vi "Corr Digitizer to Meas Folder.vi"(8 "error in":errorcluster, 10 "measurement root path":path, 11 "digitizer corr in":T1) -> (0 "error out":errorcluster, 3 "digitizer corr out":T1)   [LabVIEW 2020]
doc: "This VI will copy all digitizer corrections related folders to the measurement folder."
uses:
  Corr Digitizers.ctl
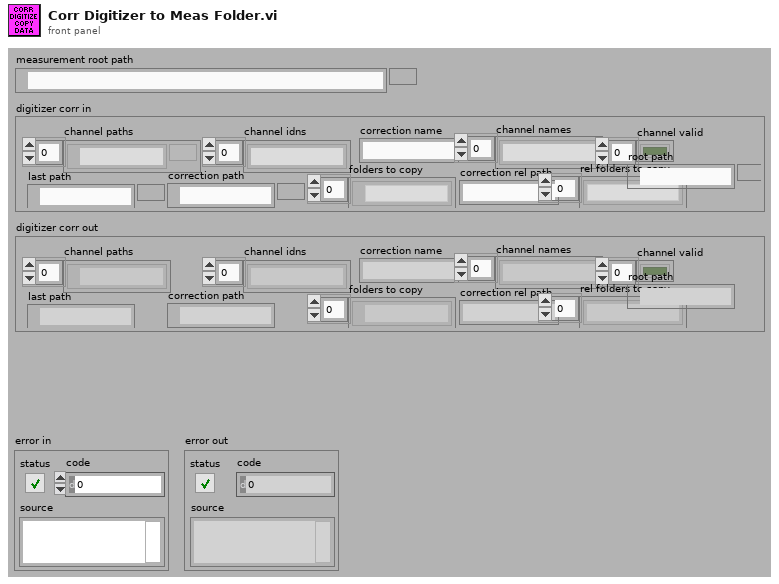
[diagram p1: front panel]
types:
  T1 = typedef "Corr Digitizers.ctl" = cluster{"last path":path, "channel paths":path[], "channel idns":string[], "correction name":string, "channel names":string[], "folders to copy":path[], "channel valid":bool[], "correction path":path, "correction rel path":string, "rel folders to copy":string[], "root path":path}
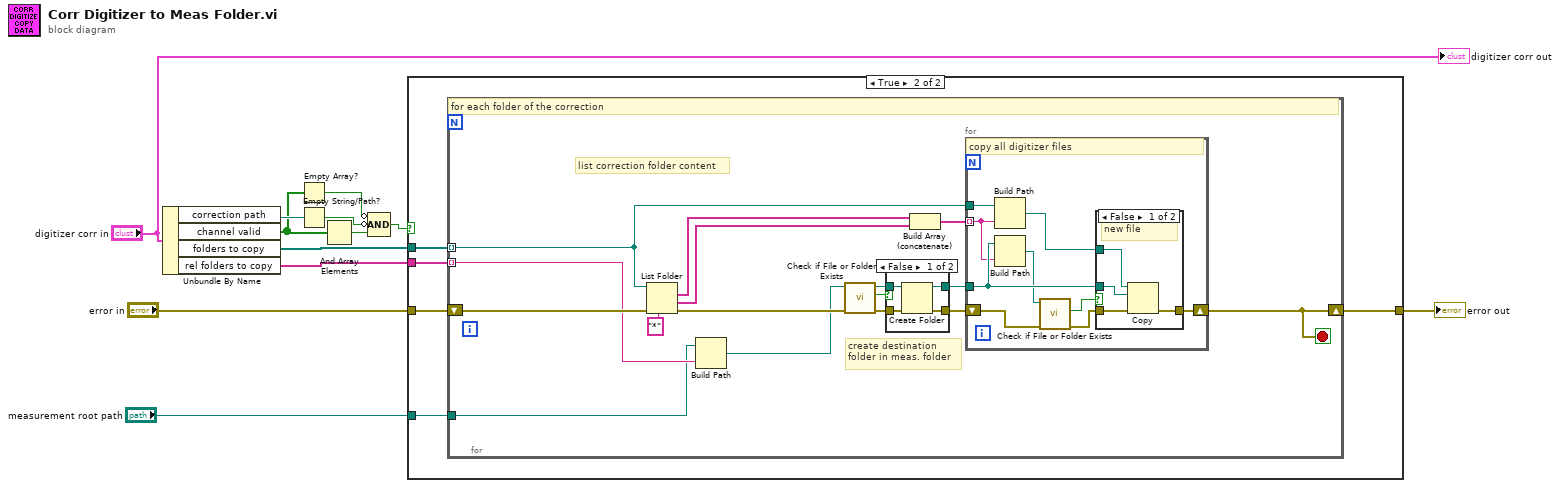
[diagram p0: block diagram]
diagram:
  n1 = Unbundle By Name("digitizer corr in") -> ("correction path"=w7:path, "channel valid"=w2:bool[], "folders to copy"=w12:path[], "rel folders to copy"=w1:string[])
  n2 = Empty Array?(array=w2) -> (empty?=w3:bool)
  n3 = Empty String/Path?(string/path=w7) -> (empty?=w5:bool)
  n4 = And Array Elements(Boolean array=w2) -> (logical AND=w6:bool)
  n5 = Compound Arithmetic op=AND(invert w3, invert w5, w6) -> (w4:bool)
  n6 = case shown="True" w4 {
    tunnel: w12 -> [_ w18]
    tunnel: "error in" -> [w13 w17]
    tunnel: [w13 w15] -> w10
    tunnel: "measurement root path" -> [_ w16]
    tunnel: w1 -> [_ w14]
    frame False {
    }
    frame True {
      n7 = for {
        tunnel: w18 -> [w22] mode=indexing
        tunnel: w16 -> [w19]
        shift-right: [w33] -> w15
        shift-left: w17 -> [w34]
        tunnel: w14 -> [w21] mode=indexing
        stop <- w33 stop-if-true
        # "create destination\nfolder in meas. folder"
        # "list correction folder content"
        # "for each folder of the correction"
        n8 = List Folder(path=w22, pattern="*", error in=w34) -> (filenames=w29:string[], folder names=w28:string[], error out=w26:errorcluster)  [unwired: 1 in, 1 out]
        n9 = Build Path(base path=w19, name or relative path=w21) -> (appended path=w20:path)
        n10 = call <vilib>:"Check if File or Folder Exists.vi"("error in (no error)"=w26, "path"=w20) -> ("error out"=w25:errorcluster, "file or folder exists?"=w23:bool, "dup path"=w24:path)  [unwired: 7 in]
        n11 = case shown="False" w23 {
          tunnel: [w38 w40] -> w31
          tunnel: [w37 w39] -> w30
          tunnel: w25 -> [w36 w40]
          tunnel: w24 -> [w35 w39]
          frame False {
            n12 = Create Folder(path (use dialog)=w35, error in=w36) -> (created path=w37:path, error out=w38:errorcluster)  [unwired: 1 in, 1 out]
          }
          frame True {
          }
        }
        n13 = Build Array (concatenate)(w29, w28) -> (w27:string[])
        n14 = for {
          tunnel: w30 -> [w45]
          shift-right: [w49] -> w33
          shift-left: w31 -> [w46]
          tunnel: w27 -> [w44] mode=indexing
          tunnel: w22 -> [w47]
          # "copy all digitizer files"
          n15 = Build Path(base path=w47, name or relative path=w44) -> (appended path=w48:path)
          n16 = Build Path(base path=w45, name or relative path=w44) -> (appended path=w43:path)
          n17 = call <vilib>:"Check if File or Folder Exists.vi"("error in (no error)"=w46, "path"=w43) -> ("error out"=w41:errorcluster, "file or folder exists?"=w42:bool)  [unwired: 7 in, 1 out]
          n18 = case shown="False" w42 {
            tunnel: w41 -> [w53 w54]
            tunnel: [w52 w54] -> w49
            tunnel: w45 -> [w51 _]
            tunnel: w48 -> [w50 _]
            frame False {
              # "new file"
              n19 = Copy(8:w53, 10:w51, 11:w50) -> (0:w52:errorcluster)  [unwired: 2 in, 2 out]
            }
            frame True {
              # "skip if file\nalready there"
            }
          }
        }
      }
    }
  }
  "error out" <- w10
  "digitizer corr out" <- "digitizer corr in"
